vi "mqtt payload to boolean.vi"(2 "boolean type":bool, 7 "String":string) -> (8 "Boolean":bool, 13 "error out":errorcluster)   [LabVIEW 2017]
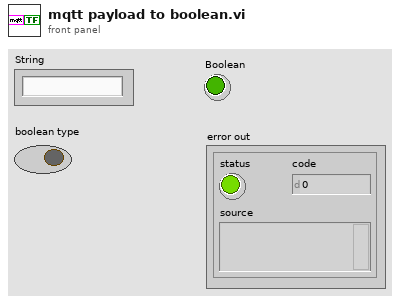
[diagram p1: front panel]
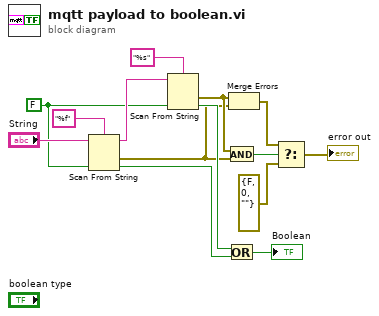
[diagram p0: block diagram]
diagram:
  w10 = FALSE ("Boolean")
  n1 = Scan From String(format string="%f", input string="String", default 1=w10) -> (remaining string=w13:string, error out=w5:errorcluster, output 1=w9:bool)  [unwired: 2 in, 1 out]
  n2 = Scan From String(format string="%s", input string=w13, default 1=w10) -> (error out=w6:errorcluster, output 1=w8:bool)  [unwired: 2 in, 2 out]
  n3 = And(x=w6, y=w5) -> (x .and. y?=w3:bool)
  n4 = Or(x=w8, y=w9) -> (x .or. y?=→"Boolean":bool)
  n5 = Merge Errors(w6, w5) -> (w2:errorcluster)
  n6 = Select(t=w2, s=w3, f=errorcluster {"status"=FALSE, "code"=0, "source"=""}) -> (s? t:f=→"error out":errorcluster)
